vi "Get Server State.vi"(8 "error in (no error)":errorcluster, 11 "OOP Query Server in":refnum<class "OOP Query Server.lvclass">) -> (0 "error out":errorcluster, 2 "Server Internal State":T1, 3 "OOP Query Server out":refnum<class "OOP Query Server.lvclass">)   [LabVIEW 2019, in "OOP Query Server.lvlib" / "OOP Query Server.lvclass"]
uses:
  OOP Query Server.lvclass
  typeDefs/Server State Data.ctl
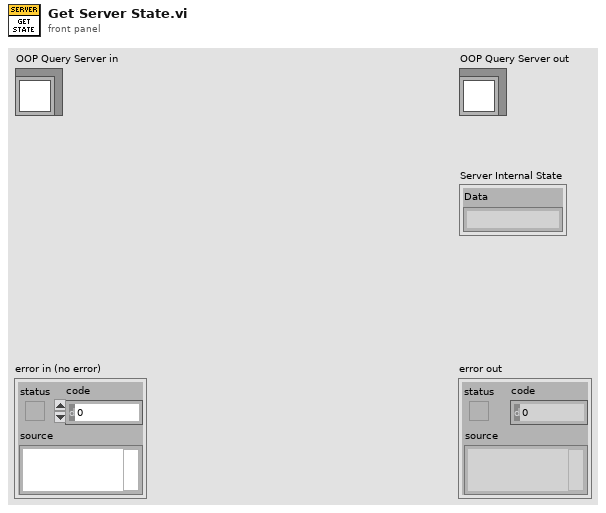
[diagram p1: front panel]
types:
  T1 = typedef "OOP Query Server.lvlib/OOP Query Server.lvclass/Server State Data.ctl" = cluster{"Data":string}
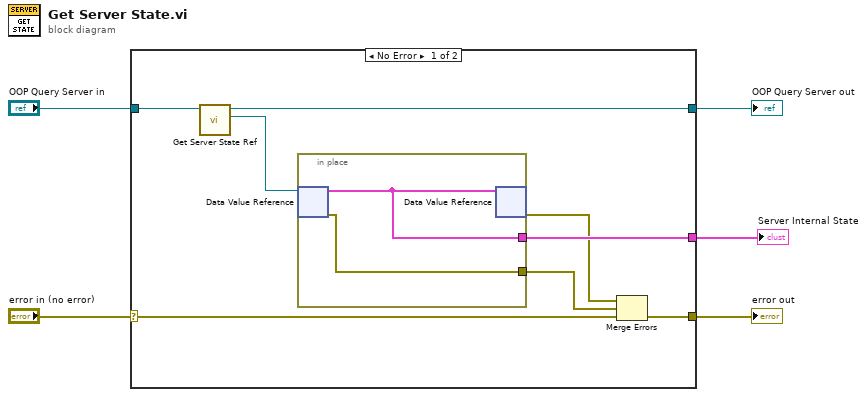
[diagram p0: block diagram]
diagram:
  n1 = case shown="No Error" "error in (no error)" {
    selector: "error in (no error)" -> [w6 w17]
    tunnel: [w8 w17] -> w4
    tunnel: [w12 w16] -> w2
    tunnel: "OOP Query Server in" -> [w13 w16]
    tunnel: [w10 _] -> w1
    frame No Error {
      n2 = call "Get Server State Ref.vi"("OOP Query Server in"=w13) -> ("Server State Ref"=w11:refnum<data-value>, "OOP Query Server out"=w12:refnum<class "OOP Query Server.lvclass">)  [unwired: 9 in]
      n3 = in-place {
        in-place-border: [w15] -> w10
        in-place-border: [w14] -> w7
        n4 = in-place-dvr #1(w11) -> (w15:T1, w14:errorcluster)
        n5 = in-place-dvr #1(w15) -> (w9:errorcluster)  [unwired: 1 out]
      }
      n6 = Merge Errors(w9, w7, w6) -> (w8:errorcluster)
    }
    frame Error {
    }
  }
  "error out" <- w4
  "OOP Query Server out" <- w2
  "Server Internal State" <- w1
